vi "brute_force.vi"() -> ()   [LabVIEW 2010]
panel:
  out "2D Array":dbl[][](array[numeric]) format="%.4f"
  in  "# of Columns":u8
  in  "# of Rows":u8
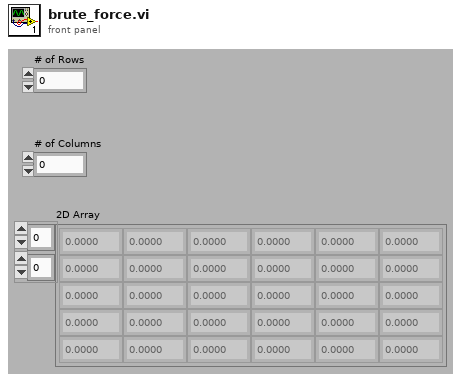
[diagram p1: front panel]
types:
  T1 = enum16{"open", "replace", "create", "open or create", "replace or create", "replace or create with confirmation"}
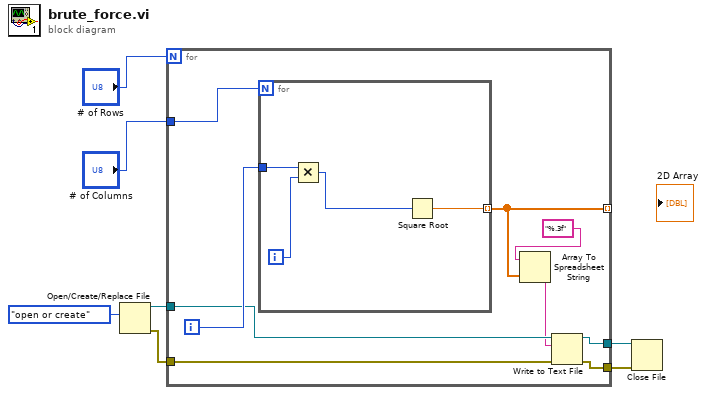
[diagram p0: block diagram]
diagram:
  n1 = Open/Create/Replace File(operation (0:open)=T1."open or create") -> (refnum out=w5:refnum<file>, error out=w3:errorcluster)  [unwired: 5 in, 1 out]
  n2 = for {
    N: "# of Rows" -> [_]
    tunnel: "# of Columns" -> [w15]
    tunnel: [w8] -> _ mode=indexing
    tunnel: w5 -> [w14]
    tunnel: [w13] -> w4
    tunnel: w3 -> [w12]
    tunnel: [w11] -> w2
    i -> [w16]
    n3 = for {
      N: w15 -> [_]
      tunnel: w16 -> [w20]
      tunnel: [w17] -> w8 mode=indexing
      i -> [w19]
      n4 = Multiply(x=w20, y=w19) -> (x*y=w18:i32)
      n5 = Square Root(x=w18) -> (sqrt(x)=w17:dbl)
    }
    n6 = Array To Spreadsheet String(array=w8, 3:"%.3f" ("format (%.3f)")) -> (spreadsheet string=w10:string)  [unwired: 1 in]
    n7 = Write to Text File(file (use dialog)=w14, text=w10, error in=w12) -> (refnum out=w13:refnum<file>, error out=w11:errorcluster)  [unwired: 1 in, 1 out]
  }
  n8 = Close File(refnum=w4, error in=w2) -> ()  [unwired: 2 out]
